vi "Init.vi"   [LabVIEW 2012]
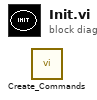
[diagram p0: block diagram]
diagram:
  n1 = call "Create_Commands.vi"() -> ()  [unwired: 1 in]
